vi "Set Sweep.vi"(0 "Sweep Name":string, 5 "Sweep in":variant, 11 "error in (no error)":errorcluster) -> (15 "error out":errorcluster)   [LabVIEW 2023, in "RFCalAndFixtureCharact.Common.lvlib"]
uses:
  RFCalAndFixtureCharact.Common.lvlib
  Type Definitions/Dictionary Operation.ctl
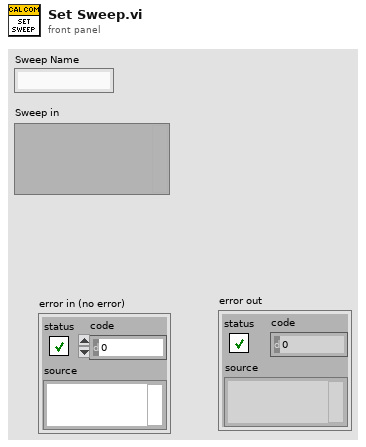
[diagram p1: front panel]
types:
  T1 = typedef "RFCalAndFixtureCharact.Common.lvlib/Dictionary Operation.ctl" = enum16{"Read", "Insert", "Remove", "Clear", "Get All", "Update"}
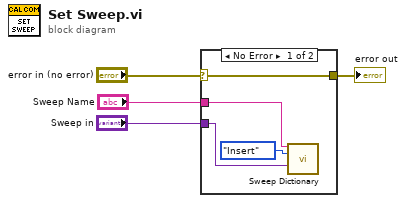
[diagram p0: block diagram]
diagram:
  n1 = case shown="No Error" "error in (no error)" {
    selector: "error in (no error)" -> [w7 w9]
    tunnel: "Sweep in" -> [w8 _]
    tunnel: [w7 w9] -> w2
    tunnel: "Sweep Name" -> [w5 _]
    frame No Error {
      n2 = call "Sweep Dictionary.vi"("Sweep name"=w5, "Action"=Dictionary_Operation."Insert", "Sweep in"=w8) -> ()  [unwired: 10 in, 3 out]
    }
    frame Error {
    }
  }
  "error out" <- w2
